vi "Smart Dashboard Data.vi"() -> ()   [LabVIEW 2014]
uses:
  2014 Dashboard Project/Vision Processing/TargetType.ctl
panel:
  out "Target Info":T2(array[cluster])
  out "Distances":T3(array[cluster])
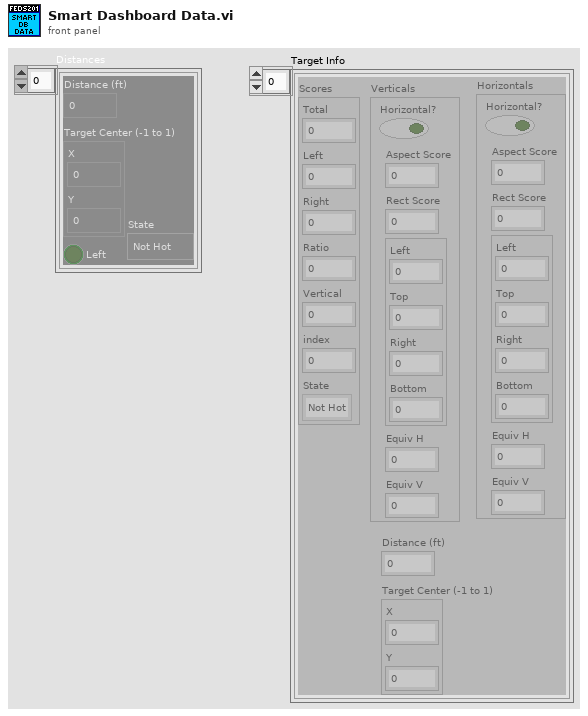
[diagram p1: front panel]
types:
  T1 = typedef "TargetType.ctl" = enum16{"Not Hot", "Hot"}
  T2 = cluster{"Scores":cluster{"Total":dbl, "Left":dbl, "Right":dbl, "Ratio":dbl, "Vertical":dbl, "index":i32, "State":T1}, "Verticals":cluster{"Horizontal?":bool, "Aspect Score":dbl, "Rect Score":dbl, cluster{"Left":dbl, "Top":dbl, "Right":dbl, "Bottom":dbl}, "Equiv H":dbl, "Equiv V":dbl}, "Horizontals":cluster{"Horizontal?":bool, "Aspect Score":dbl, "Rect Score":dbl, cluster{"Left":dbl, "Top":dbl, "Right":dbl, "Bottom":dbl}, "Equiv H":dbl, "Equiv V":dbl}, "Distance (ft)":dbl, "Target Center (-1 to 1)":cluster{"X":dbl, "Y":dbl}}[]
  T3 = cluster{"Distance (ft)":dbl, "Target Center (-1 to 1)":cluster{"X":dbl, "Y":dbl}, "Left":bool, "State":T1}[]
  T4 = cluster{"Distance (ft)":dbl, "Target Center (-1 to 1)":cluster{"X":dbl, "Y":dbl}, "Left":bool, "State":T1}
  T5 = cluster{"Scores":cluster{"Total":dbl, "Left":dbl, "Right":dbl, "Ratio":dbl, "Vertical":dbl, "index":i32, "State":T1}, "Verticals":cluster{"Horizontal?":bool, "Aspect Score":dbl, "Rect Score":dbl, cluster{"Left":dbl, "Top":dbl, "Right":dbl, "Bottom":dbl}, "Equiv H":dbl, "Equiv V":dbl}, "Horizontals":cluster{"Horizontal?":bool, "Aspect Score":dbl, "Rect Score":dbl, cluster{"Left":dbl, "Top":dbl, "Right":dbl, "Bottom":dbl}, "Equiv H":dbl, "Equiv V":dbl}, "Distance (ft)":dbl, "Target Center (-1 to 1)":cluster{"X":dbl, "Y":dbl}}
  T6 = cluster{"Total":dbl, "Left":dbl, "Right":dbl, "Ratio":dbl, "Vertical":dbl, "index":i32, "State":T1}
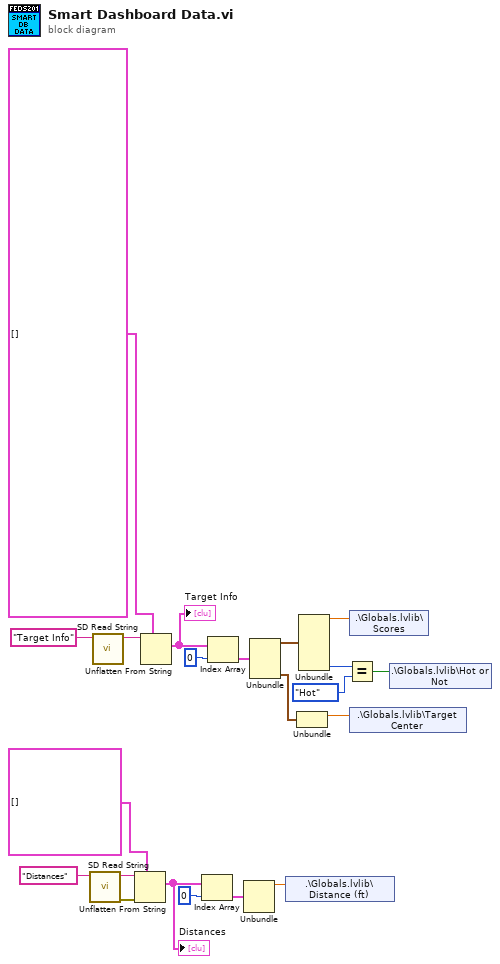
[diagram p0: block diagram]
diagram:
  n1 = call <vilib>:"SD Read String.vi"("Name"="Distances") -> ("error out"=w19:errorcluster, "String"=w18:string)  [unwired: 8 in, 1 out]
  n2 = call <vilib>:"SD Read String.vi"("Name"="Target Info") -> ("String"=w17:string)  [unwired: 8 in, 2 out]
  n3 = Unflatten From String(type=T3 [] ("Distances 2"), binary string=w18, error in (no error)=w19) -> (value=w14:T3)  [unwired: 2 in, 2 out]
  "Distances" <- w14
  n4 = Unflatten From String(type=T2 [] ("Target Info 2"), binary string=w17) -> (value=w10:T2)  [unwired: 3 in, 2 out]
  "Target Info" <- w10
  n5 = Index Array(array=w14, index=0) -> (element=w12:T4)
  n6 = Index Array(array=w10, index=0) -> (element=w8:T5)
  n7 = Unbundle(w12) -> ("Distance (ft)"=w11:dbl)  [unwired: 3 out]
  n8 = Unbundle(w8) -> ("Scores"=w7:T6, "Target Center (-1 to 1)"=w4:cluster{"X":dbl, "Y":dbl})  [unwired: 3 out]
  n9 = shared-variable ".\\Globals.lvlib\\Distance (ft)"(w11) -> ()  [unwired: 1 in, 1 out]
  n10 = Unbundle(w4) -> ("X"=w5:dbl)  [unwired: 1 out]
  n11 = Unbundle(w7) -> ("Total"=w6:dbl, "State"=w3:T1)  [unwired: 5 out]
  n12 = Equal?(x=w3, y=TargetType."Hot") -> (x = y?=w1:bool)
  n13 = shared-variable ".\\Globals.lvlib\\Scores"(w6) -> ()  [unwired: 1 in, 1 out]
  n14 = shared-variable ".\\Globals.lvlib\\Target Center"(w5) -> ()  [unwired: 1 in, 1 out]
  n15 = shared-variable ".\\Globals.lvlib\\Hot or Not"(w1) -> ()  [unwired: 1 in, 1 out]
